vi "Get all Dependencies.vi"(0 "Measurement paths":path[](array[path]), 11 "error in (no error)":errorcluster) -> (4 "All dependencies":path[][](array[path]), 6 "Instrument containing subVIs":path[][](array[path]), 15 "error out":errorcluster)   [LabVIEW 2021]
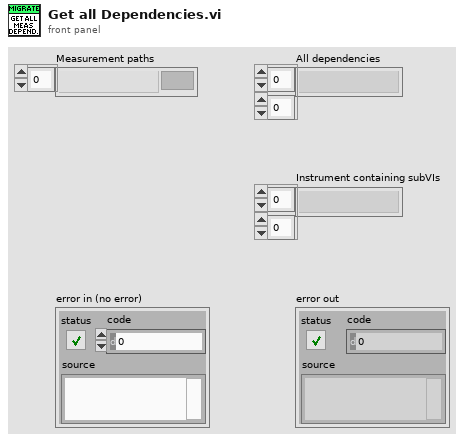
[diagram p1: front panel]
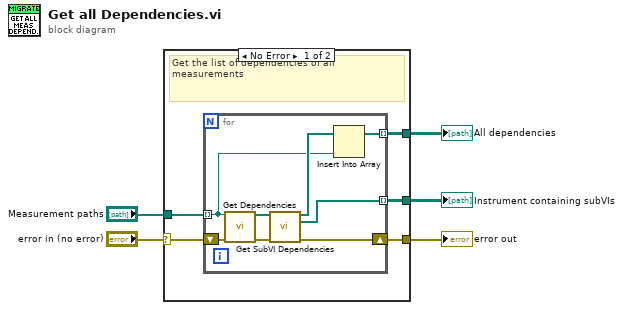
[diagram p0: block diagram]
diagram:
  n1 = case shown="No Error" "error in (no error)" {
    selector: "error in (no error)" -> [w7 w19]
    tunnel: "Measurement paths" -> [w10 _]
    tunnel: [w9 _] -> w4
    tunnel: [w8 w19] -> w3
    tunnel: [w6 _] -> w1
    frame No Error {
      # "Get the list of dependencies of all measurements"
      n2 = for {
        shift-right: [w16] -> w8
        shift-left: w7 -> [w18]
        tunnel: w10 -> [w11] mode=indexing
        tunnel: [w12] -> w9 mode=indexing
        tunnel: [w14] -> w6 mode=indexing
        n3 = call "Get Dependencies.vi"("VI path"=w11, "error in (no error)"=w18) -> ("Existing dependencies"=w15:path[], "error out"=w17:errorcluster)  [unwired: 12 in]
        n4 = call "Get SubVI Dependencies.vi"("Dependency Paths"=w15, "error in (no error)"=w17) -> ("All dependencies"=w13:path[], "Instrument containing subVIs"=w14:path[], "error out"=w16:errorcluster)  [unwired: 11 in]
        n5 = Insert Into Array(array=w13, new element=w11) -> (w12:path[])  [unwired: 1 in]
      }
    }
    frame Error {
      # "Pass"
    }
  }
  "All dependencies" <- w4
  "error out" <- w3
  "Instrument containing subVIs" <- w1
